vi "UT_007_Edit TOML data.vi"   [LabVIEW 2020]
uses:
  <vilib>/addons/_JKI Toolkits/Caraya/classes/Assert/Assert True.vi
  <vilib>/addons/_JKI Toolkits/Caraya/classes/Test/Test.lvclass
  <vilib>/addons/_JKI Toolkits/Caraya/classes/Assert/Assert.lvclass
  lib/TOML.lvlib
types:
  T1 = cluster{"cluster":cluster{"string":string, "bool":bool, "path":path}, "1d-array-cluster":cluster{"string":string, "int":i32}[]}
  T2 = cluster{"string":string, "bool":bool, "path":path}
  T3 = typedef "TOML.lvlib/TOML Value.ctl" = cluster{"type":enum16{"Table", "Array", "String", "Integer", "Float", "Boolean", "Offset Date-Time", "Local Date-Time", "Local Date", "Local Time", "Path"}, "value":variant}
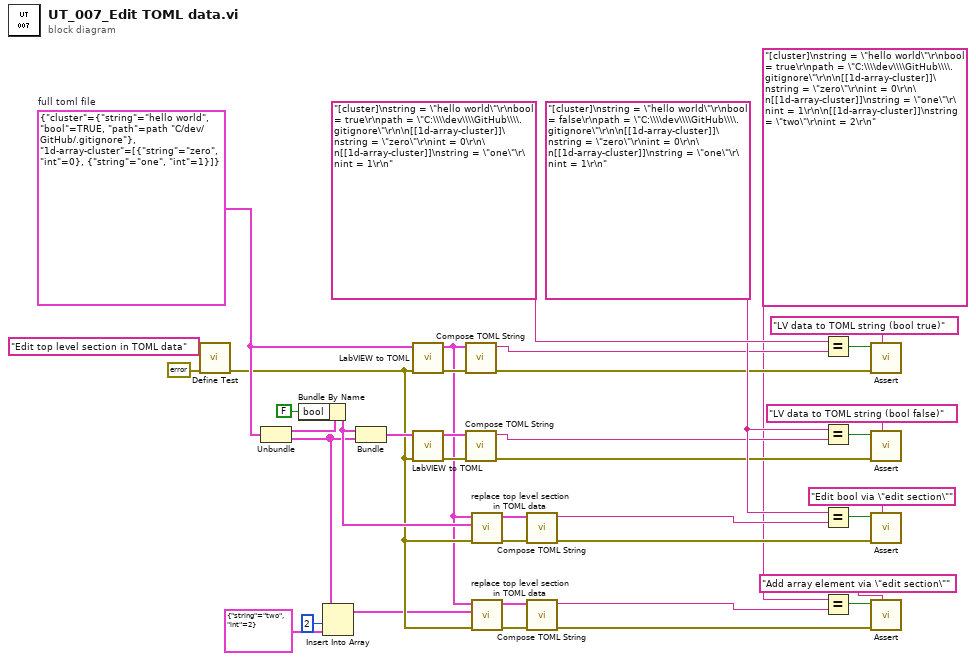
[diagram p0: block diagram]
diagram:
  w23 = "[cluster]\nstring = \"hello world\"\r\nbool = false\r\npath = \"C:\\\\dev\\\\GitHub\\\\.gitignore\"\r\n\n[[1d-array-cluster]]\nstring = \"zero\"\r\nint = 0\r\n\n[[1d-array-cluster]]\nstring = \"one\"\r\nint = 1\r\n" ("x")
  w30 = T1 {"cluster"={"string"="hello world", "bool"=TRUE, "path"=path "C:/dev/GitHub/.gitignore"}, "1d-array-cluster"=[{"string"="zero", "int"=0}, {"string"="one", "int"=1}]}  # full toml file
  n1 = call <vilib>:"Define Test.vi"("error in (no error)"=errorcluster {"status"=FALSE, "code"=0, "source"=""}, "Label (VI Title)"="Edit top level section in TOML data") -> ("error out"=w8:errorcluster)  [unwired: 8 in, 1 out]
  n2 = Unbundle(w30) -> ("cluster"=w7:T2, "1d-array-cluster"=w6:cluster{"string":string, "int":i32}[])
  n3 = Bundle By Name(cluster=w7, "bool"=FALSE) -> (w15:T2)
  n4 = Insert Into Array(array=w6, index=2, new element=cluster{"string":string, "int":i32} {"string"="two", "int"=2}) -> (w3:cluster{"string":string, "int":i32}[])
  n5 = Bundle("cluster"=w15, "1d-array-cluster"=w6) -> (w28:T1)  [unwired: 1 in]
  n6 = call "LabVIEW to TOML.vi"("error in (no error)"=w8, "LV Value"=w30) -> ("error out"=w22:errorcluster, "TOML Value"=w5:T3)  [unwired: 7 in, 1 out]
  n7 = call "LabVIEW to TOML.vi"("error in (no error)"=w8, "LV Value"=w28) -> ("error out"=w19:errorcluster, "TOML Value"=w20:T3)  [unwired: 7 in, 1 out]
  n8 = call "Compose TOML String.vi"("error in (no error)"=w22, "Value"=w5) -> ("error out"=w21:errorcluster, "String"=w16:string)  [unwired: 8 in]
  n9 = call "Compose TOML String.vi"("error in (no error)"=w19, "Value"=w20) -> ("error out"=w18:errorcluster, "String"=w17:string)  [unwired: 8 in]
  n10 = call "replace top level section in TOML data.vi"("error in (no error)"=w8, "Section data"=w15, "Value in"=w5) -> ("error out"=w35:errorcluster, "Value out"=w33:T3)  [unwired: 7 in]
  n11 = call "replace top level section in TOML data.vi"("error in (no error)"=w8, "Section data"=w3, "Value in"=w5) -> ("error out"=w10:errorcluster, "Value out"=w12:T3)  [unwired: 7 in]
  n12 = call "Compose TOML String.vi"("error in (no error)"=w35, "Value"=w33) -> ("error out"=w34:errorcluster, "String"=w24:string)  [unwired: 8 in]
  n13 = call "Compose TOML String.vi"("error in (no error)"=w10, "Value"=w12) -> ("error out"=w11:errorcluster, "String"=w14:string)  [unwired: 8 in]
  n14 = Equal?(x="[cluster]\nstring = \"hello world\"\r\nbool = true\r\npath = \"C:\\\\dev\\\\GitHub\\\\.gitignore\"\r\n\n[[1d-array-cluster]]\nstring = \"zero\"\r\nint = 0\r\n\n[[1d-array-cluster]]\nstring = \"one\"\r\nint = 1\r\n", y=w16) -> (x = y?=w31:bool)
  n15 = Equal?(x=w23, y=w17) -> (x = y?=w26:bool)
  n16 = Equal?(x=w23, y=w24) -> (x = y?=w25:bool)
  n17 = Equal?(x="[cluster]\nstring = \"hello world\"\r\nbool = true\r\npath = \"C:\\\\dev\\\\GitHub\\\\.gitignore\"\r\n\n[[1d-array-cluster]]\nstring = \"zero\"\r\nint = 0\r\n\n[[1d-array-cluster]]\nstring = \"one\"\r\nint = 1\r\n\n[[1d-array-cluster]]\nstring = \"two\"\r\nint = 2\r\n", y=w14) -> (x = y?=w13:bool)
  n18 = call-poly <vilib>:"Assert.vi"("Label"="LV data to TOML string (bool true)" ("Label (VI Title)"), "error in (no error)"=w21, "True?"=w31) -> ()  [unwired: 7 in, 2 out]
  n19 = call-poly <vilib>:"Assert.vi"("Label"="LV data to TOML string (bool false)" ("Label (VI Title)"), "error in (no error)"=w18, "True?"=w26) -> ()  [unwired: 7 in, 2 out]
  n20 = call-poly <vilib>:"Assert.vi"("Label"="Edit bool via \"edit section\"" ("Label (VI Title)"), "error in (no error)"=w34, "True?"=w25) -> ()  [unwired: 7 in, 2 out]
  n21 = call-poly <vilib>:"Assert.vi"("Label"="Add array element via \"edit section\"" ("Label (VI Title)"), "error in (no error)"=w11, "True?"=w13) -> ()  [unwired: 7 in, 2 out]
